vi "test-UKF-GetDynamics.vi"(9 "U":T1, 10 "X":T1, 11 "Variant":variant) -> (0 "Error":bool, 3 "Return":T1)   [LabVIEW 2019]
uses:
  <vilib>/Analysis/Matrix/Datatypes/RealMatrix.ctl
  <vilib>/Rock Robotics/WPI/ThirdParty/JAS_Junk/TrajLib/DCMotor_New.vi
  <vilib>/Rock Robotics/WPI/ThirdParty/JAS_Junk/TrajLib/Units_RotationsPerMinuteToRadiansPerSecond.vi
  <vilib>/Rock Robotics/WPI/ThirdParty/JAS_Junk/TrajLib/MatBuilder_Create.vi
  <vilib>/Rock Robotics/WPI/ThirdParty/JAS_Junk/TrajLib/Trajectory_Library.lvlib
  <vilib>/Analysis/Matrix/NI_Matrix.lvlib
panel:
  # "6, 1"
  # "2, 1"
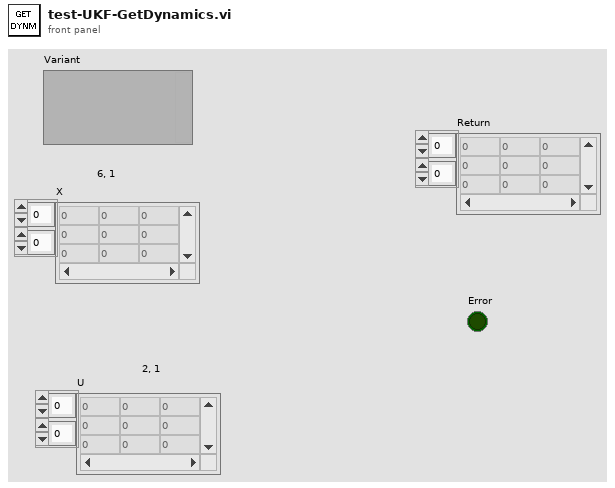
[diagram p1: front panel]
types:
  T1 = typedef "NI_Matrix.lvlib/RealMatrix.ctl" = dbl[][]
  T2 = typedef "Trajectory_Library.lvlib/DCMOTOR.CTL" = cluster{"nominalVoltage_Volts":dbl, "StallTorque_NM":dbl, "StallCurrent_Amps":dbl, "FreeCurrent_Amps":dbl, "FreeSpeed_RadPerSec":dbl, "R_Ohms":dbl, "KvINV_RadPerSecPerVolt":dbl, "Kt_NMPerAmp":dbl, "L_H":dbl, "Jr_KgM2":dbl}
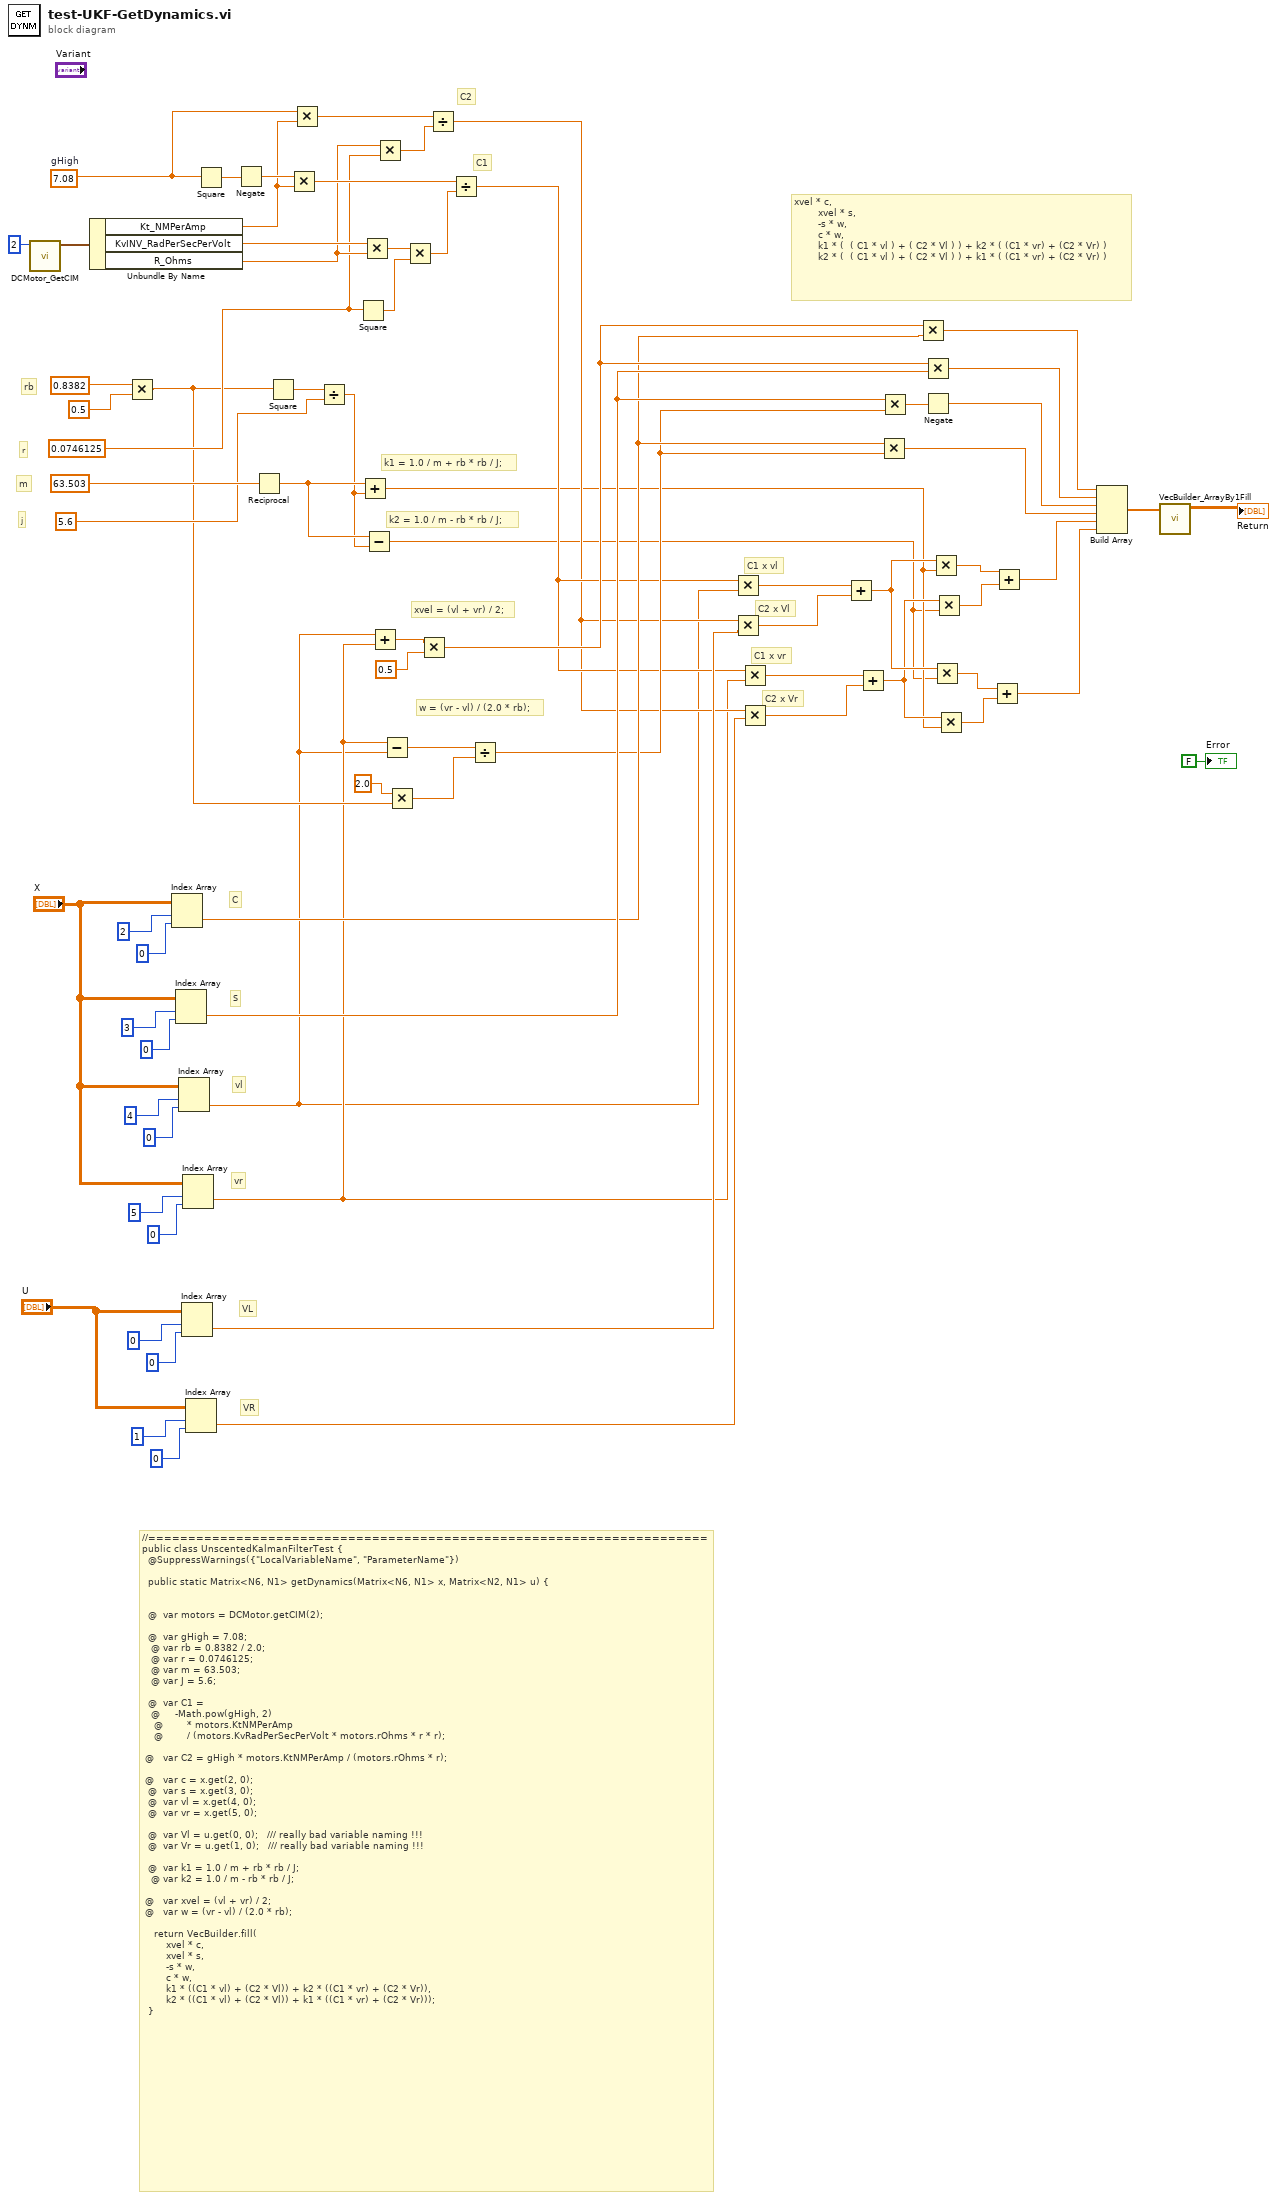
[diagram p0: block diagram]
diagram:
  w60 = 0.0746125
  w63 = 7.08  # gHigh
  # "C2 x Vr"
  # "C1 x vr"
  # "C2 x Vl"
  # "C1 x vl"
  # "xvel * c,\n        xvel * s,\n        -s * w,\n        c * w,\n        k1 * (  ( C1 * vl ) + ( C2 * Vl ) ) + k2 * ( (C1 * vr) + (C2 * Vr) )\n        k2 * (  ( C1 * vl ) + ( C2 * Vl ) ) + k1 * ( (C1 * vr) + (C2 * Vr) )"
  # "w = (vr - vl) / (2.0 * rb);"
  # "xvel = (vl + vr) / 2;"
  # "k2 = 1.0 / m - rb * rb / J;"
  # "k1 = 1.0 / m + rb * rb / J;"
  # "VR"
  # "VL"
  # "vr"
  # "vl"
  # "S"
  # "C"
  # "C2"
  # "C1"
  # "j"
  # "m"
  # "r"
  # "rb"
  # "//======================================================================\npublic class UnscentedKalmanFilterTest {\n  @SuppressWarnings({\"LocalVariableName\", \"ParameterName\"})\n\n  public static Matrix<N6, N1> getDynamics(Matrix<N6, N1> x, Matrix<N2, N1> u) {\n\n\n  @  var motors = DCMotor.getCIM(2);\n\n  @  var gHigh = 7.08;\n   @ var rb = 0.8382 / 2.0;\n   @ var r = 0.0746125;\n   @ var m = 63.503;\n   @ var J = 5.6;\n\n  @  var C1 =\n   @     -Math.pow(gHigh, 2)\n    @        * motors.KtNMPerAmp\n    @        / (motors.KvRadPerSecPerVolt * motors.rOhms * r * r);\n\n @   var C2 = gHigh * motors.KtNMPerAmp / (motors.rOhms * r);\n\n @   var c = x.get(2, 0);\n  @  var s = x.get(3, 0);\n  @  var vl = x.get(4, 0);\n  @  var vr = x.get(5, 0);\n\n  @  var Vl = u.get(0, 0);   /// really bad variable naming !!!\n  @  var Vr = u.get(1, 0);   /// really bad variable naming !!!\n\n  @  var k1 = 1.0 / m + rb * rb / J;\n   @ var k2 = 1.0 / m - rb * rb / J;\n\n @   var xvel = (vl + vr) / 2;\n @   var w = (vr - vl) / (2.0 * rb);\n\n    return VecBuilder.fill(\n        xvel * c,\n        xvel * s,\n        -s * w,\n        c * w,\n        k1 * ((C1 * vl) + (C2 * Vl)) + k2 * ((C1 * vr) + (C2 * Vr)),\n        k2 * ((C1 * vl) + (C2 * Vl)) + k1 * ((C1 * vr) + (C2 * Vr)));\n  }"
  n1 = call <vilib>:"DCMotor_GetCIM.vi"("Num Motors"=2) -> ("DCMOTOR"=w70:T2)  [unwired: 10 in]
  n2 = Unbundle By Name(w70) -> ("Kt_NMPerAmp"=w62:dbl, "KvINV_RadPerSecPerVolt"=w68:dbl, "R_Ohms"=w61:dbl)
  n3 = Multiply(x=0.8382, y=0.5) -> (x*y=w34:dbl)
  n4 = Index Array(array="X", index (row)=2, index (col)=0) -> (element=w28:dbl)
  n5 = Index Array(array="X", index (row)=3, index (col)=0) -> (element=w29:dbl)
  n6 = Index Array(array="X", index (row)=4, index (col)=0) -> (element=w1:dbl)
  n7 = Index Array(array="U", index (row)=0, index (col)=0) -> (element=w21:dbl)
  n8 = Index Array(array="X", index (row)=5, index (col)=0) -> (element=w2:dbl)
  n9 = Index Array(array="U", index (row)=1, index (col)=0) -> (element=w18:dbl)
  n10 = Square(x=w63) -> (x^2=w71:dbl)
  n11 = Negate(x=w71) -> (-x=w69:dbl)
  n12 = Reciprocal(x=63.503) -> (1/x=w39:dbl)
  n13 = Square(x=w34) -> (x^2=w41:dbl)
  n14 = Multiply(x=w69, y=w62) -> (x*y=w65:dbl)
  n15 = Multiply(x=w63, y=w62) -> (x*y=w59:dbl)
  n16 = Divide(x=w41, y=5.6) -> (x/y=w38:dbl)
  n17 = Square(x=w60) -> (x^2=w66:dbl)
  n18 = Add(x=w39, y=w38) -> (x+y=w11:dbl)
  n19 = Multiply(x=w68, y=w61) -> (x*y=w67:dbl)
  n20 = Subtract(x=w39, y=w38) -> (x-y=w10:dbl)
  n21 = Add(x=w1, y=w2) -> (x+y=w37:dbl)
  n22 = Multiply(x=w61, y=w60) -> (x*y=w58:dbl)
  n23 = Subtract(x=w2, y=w1) -> (x-y=w33:dbl)
  n24 = Multiply(x=2.0, y=w34) -> (x*y=w32:dbl)
  n25 = Multiply(x=w67, y=w66) -> (x*y=w64:dbl)
  n26 = Multiply(x=w37, y=0.5) -> (x*y=w31:dbl)
  n27 = Divide(x=w59, y=w58) -> (x/y=w19:dbl)
  n28 = Divide(x=w65, y=w64) -> (x/y=w20:dbl)
  n29 = Divide(x=w33, y=w32) -> (x/y=w27:dbl)
  n30 = Multiply(x=w20, y=w1) -> (x*y=w17:dbl)
  n31 = Multiply(x=w19, y=w21) -> (x*y=w16:dbl)
  n32 = Multiply(x=w20, y=w2) -> (x*y=w15:dbl)
  n33 = Multiply(x=w19, y=w18) -> (x*y=w14:dbl)
  n34 = Add(x=w17, y=w16) -> (x+y=w13:dbl)
  n35 = Add(x=w15, y=w14) -> (x+y=w12:dbl)
  n36 = Multiply(x=w28, y=w27) -> (x*y=w23:dbl)
  n37 = Multiply(x=w29, y=w27) -> (x*y=w30:dbl)
  n38 = Multiply(x=w31, y=w28) -> (x*y=w26:dbl)
  n39 = Multiply(x=w31, y=w29) -> (x*y=w25:dbl)
  n40 = Negate(x=w30) -> (-x=w24:dbl)
  n41 = Multiply(x=w13, y=w11) -> (x*y=w9:dbl)
  n42 = Multiply(x=w13, y=w10) -> (x*y=w5:dbl)
  n43 = Multiply(x=w12, y=w10) -> (x*y=w8:dbl)
  n44 = Multiply(x=w12, y=w11) -> (x*y=w7:dbl)
  n45 = Add(x=w5, y=w7) -> (x+y=w4:dbl)
  n46 = Add(x=w9, y=w8) -> (x+y=w6:dbl)
  n47 = Build Array(w26, w25, w24, w23, w6, w4) -> (w22:dbl[])
  n48 = call <vilib>:"VecBuilder_ArrayBy1Fill.vi"("R Array"=w22) -> ("Output Vector"=→"Return":T1)  [unwired: 10 in]
  "Error" <- FALSE ("Error")
